vi "Start Sequential Monitor if Not Started.vi"(8 "error in":errorcluster, 11 "core handle in":u64) -> (0 "error out":errorcluster, 3 "core handle out":u64)   [LabVIEW 2020, in "Ballard ARINC 429 Engine.lvlib" / "Custom Device.lvlib"]
uses:
  Custom Device.lvlib
  <instrlib>/BTICardLib/BTICardLV.lvlib
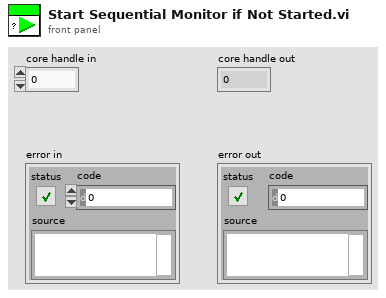
[diagram p1: front panel]
types:
  T1 = typedef "BTICardLV.lvlib/Seq Run Status.ctl" = u32
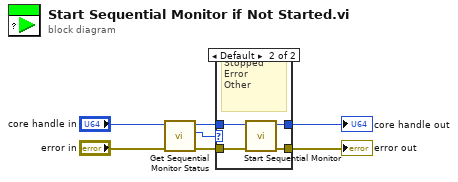
[diagram p0: block diagram]
diagram:
  n1 = call <instrlib>:"Get Sequential Monitor Status.vi"("error in (no error)"="error in", "core handle in"="core handle in") -> ("error out"=w4:errorcluster, "run status"=w5:T1, "core handle out"=w7:u64)  [unwired: 6 in, 1 out]
  n2 = case shown="Default" w5 {
    tunnel: w4 -> [w9 w13]
    tunnel: [w9 w12] -> w2
    tunnel: w7 -> [w8 w11]
    tunnel: [w8 w10] -> w1
    frame 0 {
      # "Started"
    }
    frame Default {
      # "Stopped\nError\nOther"
      n3 = call <instrlib>:"Start Sequential Monitor.vi"("error in (no error)"=w13, "core handle in"=w11) -> ("error out"=w12:errorcluster, "core handle out"=w10:u64)  [unwired: 8 in]
    }
  }
  "error out" <- w2
  "core handle out" <- w1
